vi "WriteIniKey.vi"(7 "Section Name":string, 8 "Key Val In":dbl, 9 "?":T2=enum."Read Key", 10 "Key Name":string, 11 "Ini File Refnum":T1) -> (3 "Key Val Out":dbl)   [LabVIEW 2014]
uses:
  ReadWriteIniKey.ctl
  <vilib>/Utility/config.llb/Config Data RefNum.ctl
  <vilib>/Utility/config.llb/Write Key (Double).vi
  <vilib>/Utility/config.llb/Read Key (Double).vi
  <vilib>/Utility/config.llb/NI_LVConfig.lvlib
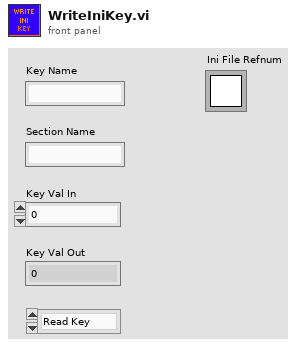
[diagram p1: front panel]
types:
  T1 = typedef "NI_LVConfig.lvlib/Config Data RefNum.ctl" = refnum<k1>
  T2 = typedef "ReadWriteIniKey.ctl" = enum16{"Write Key", "Read Key"}
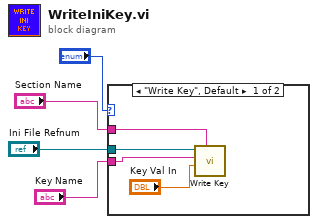
[diagram p0: block diagram]
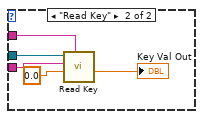
[diagram p2: hidden frame]
diagram:
  n1 = case shown="\"Write Key\", Default" "?" {
    tunnel: "Section Name" -> [w8 w13]
    tunnel: "Key Name" -> [w7 w12]
    tunnel: "Ini File Refnum" -> [w5 w9]
    frame "Write Key", Default {
      n2 = call-poly <vilib>:"Write Key.vi"("section"=w8, "value"="Key Val In", "key"=w7, "refnum"=w5) -> ()  [unwired: 5 in, 3 out]
    }
    frame "Read Key" {
      n3 = call-poly <vilib>:"Read Key.vi"("section"=w13, "default value"=0.0, "key"=w12, "refnum"=w9) -> ("value"=→"Key Val Out":dbl)  [unwired: 4 in, 3 out]
    }
  }
